vi "Result_Test.vi"(8 "error in (no error)":errorcluster caption="entrée d'erreur (pas d'erreur)", 11 "Get_Voltage en entrée":refnum<class "Nodon_Set_ZCR_Calibration.lvclass">) -> (0 "error out":errorcluster caption="sortie d'erreur", 3 "Get_Voltage en sortie":refnum<class "Nodon_Set_ZCR_Calibration.lvclass">)   [LabVIEW 2020, in "Library Test.lvlib" / "Nodon_Set_ZCR_Calibration.lvclass"]
uses:
  Nodon_Set_ZCR_Calibration.lvclass
  Nodon_Send_Command_UART/Nodon_Send_Command_UART.lvclass
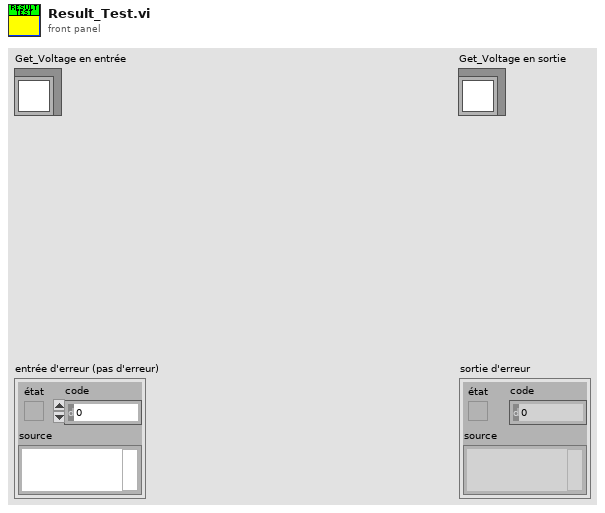
[diagram p1: front panel]
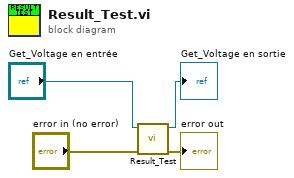
[diagram p0: block diagram]
diagram:
  n1 = call-parent "Result_Test.vi"("error in (no error)"="error in (no error)", "Get_Voltage en entrée"="Get_Voltage en entrée") -> ("error out"=→"error out":errorcluster, "Get_Voltage en sortie"=→"Get_Voltage en sortie":refnum<class "Nodon_Set_ZCR_Calibration.lvclass">)  [unwired: 8 in]
